vi "half_wave_selection.vi"(6 "signal in":waveform(dbl), 9 "data":waveform(dbl), 10 "Numeric":dbl, 11 "frequency":dbl) -> (1 "waveform out":waveform(dbl), 2 "waveform out 2":waveform(dbl), 3 "waveform out 3":waveform(dbl))   [LabVIEW 2019]
uses:
  <vilib>/Waveform/WDTOps.llb/WDT Get Waveform Subset DBL.vi
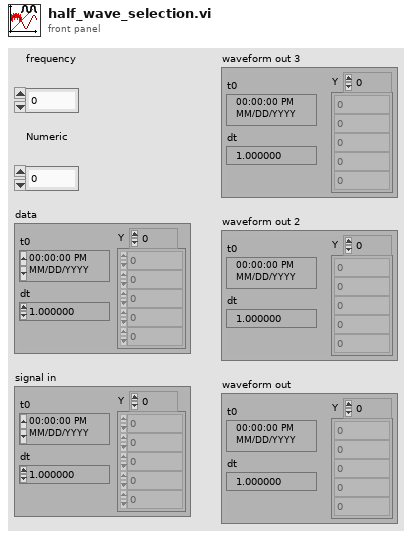
[diagram p1: front panel]
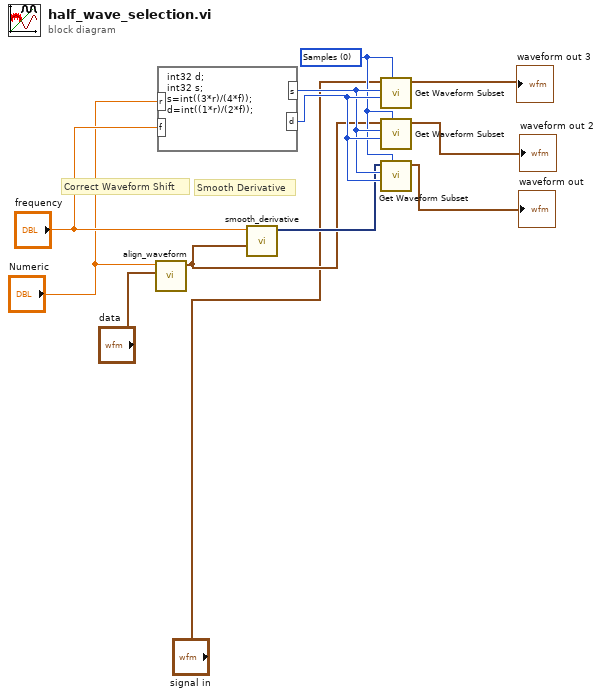
[diagram p0: block diagram]
diagram:
  w7 = u16 0 items=["Samples", "Relative Time"] ("start/duration format")
  # "Smooth Derivative"
  # "Correct Waveform Shift"
  n1 = call "align_waveform.vi"("Input Waveform"="data", "Sample Rate to be Wired"="Numeric") -> ("Output Waveform"=w5:waveform(dbl))  [unwired: 9 in]
  n2 = formula code="int32 d;\nint32 s;\ns=int((3*r)/(4*f));\nd=int((1*r)/(2*f));"("f"="frequency", "r"="Numeric") -> ("d"=w9:i32, "s"=w8:i32)
  n3 = call "smooth_derivative.vi"("Output Waveform"=w5, "frequency"="frequency") -> ("Filtered Signal"=w6:dynamicdata)  [unwired: 9 in]
  n4 = call-poly <vilib>:"Get Waveform Subset.vi"("start/duration format"=w7, "duration"=w9, "start samples/time"=w8, "waveform in"="signal in") -> ("waveform out"=→"waveform out 3":waveform(dbl))  [unwired: 2 in, 3 out]
  n5 = call-poly <vilib>:"Get Waveform Subset.vi"("start/duration format"=w7, "duration"=w9, "start samples/time"=w8, "waveform in"=w5) -> ("waveform out"=→"waveform out 2":waveform(dbl))  [unwired: 2 in, 3 out]
  n6 = call-poly <vilib>:"Get Waveform Subset.vi"("start/duration format"=w7, "duration"=w9, "start samples/time"=w8, "waveform in"=w6) -> ("waveform out"=→"waveform out":waveform(dbl))  [unwired: 2 in, 3 out]
